vi "Read Current.vi"(8 "error in (no error)":errorcluster, 11 "PathTokenizer in":refnum<class "PathTokenizer.lvclass">) -> (0 "error out":errorcluster, 2 "Current":i32, 3 "PathTokenizer out":refnum<class "PathTokenizer.lvclass">)   [LabVIEW 2019, in "PathTokenizer.lvclass"]
uses:
  PathTokenizer.lvclass
  PathTokenizer.lvclass/PathTokenizer.ctl
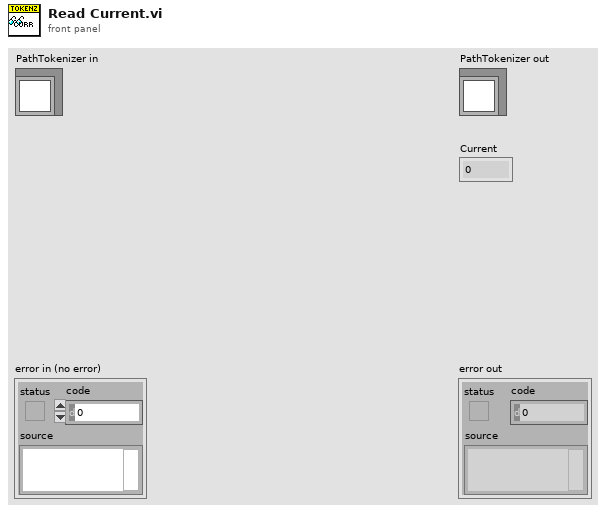
[diagram p1: front panel]
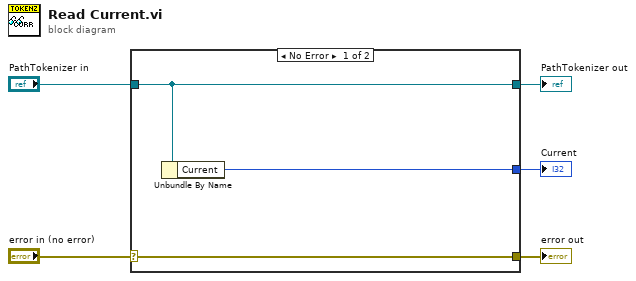
[diagram p0: block diagram]
diagram:
  n1 = case shown="No Error" "error in (no error)" {
    selector: "error in (no error)" -> [w8 w9]
    tunnel: [w8 w9] -> w4
    tunnel: [w7 w10] -> w2
    tunnel: "PathTokenizer in" -> [w7 w10]
    tunnel: [w6 _] -> w1
    frame No Error {
      n2 = Unbundle By Name(w7) -> ("Current"=w6:i32)
    }
    frame Error {
    }
  }
  "error out" <- w4
  "PathTokenizer out" <- w2
  "Current" <- w1
